vi "FindShift.vi"(9 "SMPS Sizes":dbl[](array[numeric]), 10 "Concentration":dbl[](array[numeric]), 11 "Sizes":dbl) -> (1 "Peak Center":dbl, 2 "Shift in nm":dbl, 3 "Shift in Log scale":dbl)   [LabVIEW 2013]
doc: "Finds the size shift of the smpls multiple charge correction file relative to the actual selected sizes"
uses:
  <vilib>/Analysis/NI_AALPro.lvlib
panel:
  out "Simplex 2":cluster{dbl[], dbl[]}(graph)
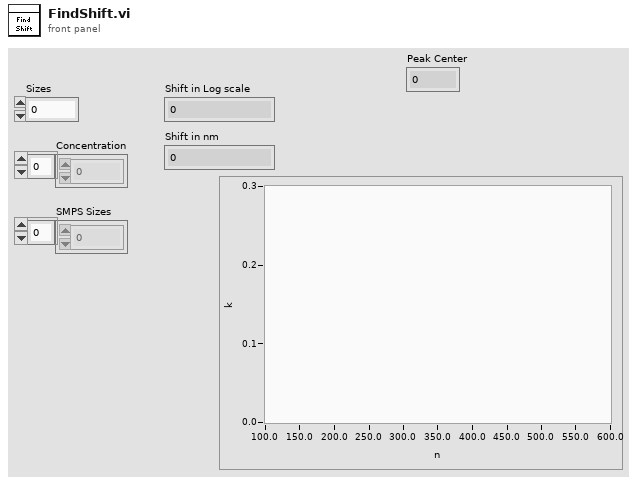
[diagram p1: front panel]
types:
  T1 = cluster{"SMPS Sizes":dbl[], "Concentration":dbl[]}
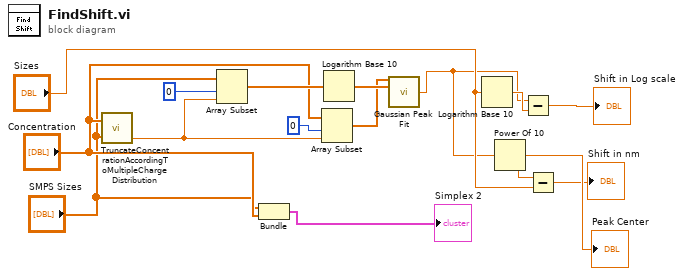
[diagram p0: block diagram]
diagram:
  n1 = call "TruncateConcentrationAccordingToMultipleChargeDistribution.vi"("Concentration"="Concentration", "Sizes"="SMPS Sizes") -> ("Location"=w12:dbl)  [unwired: 2 out]
  n2 = Array Subset(array="SMPS Sizes", index=0, length=w12) -> (w9:dbl[])
  n3 = Bundle("SMPS Sizes"="SMPS Sizes", "Concentration"="Concentration") -> (→"Simplex 2":T1)  [unwired: 1 in]
  n4 = Array Subset(array="Concentration", index=0, length=w12) -> (w8:dbl[])
  n5 = Logarithm Base 10(1:w9) -> (0:w13:dbl[])
  n6 = call <vilib>:"Gaussian Peak Fit.vi"("Y"=w8, "X"=w13) -> ("center"=w5:dbl)  [unwired: 7 in, 6 out]
  n7 = Logarithm Base 10(1:"Sizes") -> (0:w14:dbl)
  n8 = Power Of 10(x=w5) -> (10^x=w4:dbl)
  "Peak Center" <- w4
  n9 = Subtract(x=w5, y=w14) -> (x-y=→"Shift in Log scale":dbl)
  n10 = Subtract(x=w4, y="Sizes") -> (x-y=→"Shift in nm":dbl)
